vi "Print.vi"(11 "Printer In":refnum<class "Printer.lvclass">) -> (3 "Printer Out":refnum<class "Printer.lvclass">)   [LabVIEW 2018, in "Printer.lvclass"]
uses:
  Printer.lvclass
  IPrinter/IPrinter.lvclass
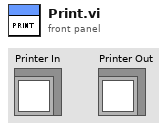
[diagram p1: front panel]
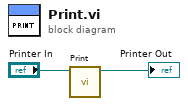
[diagram p0: block diagram]
diagram:
  n1 = call-parent "Print.vi"("IPrinter In"="Printer In") -> ("IPrinter Out"=→"Printer Out":refnum<class "Printer.lvclass">)  [unwired: 10 in]
